vi "SaveDeviceHeader.vi"(0 "File Refnum in":refnum<file>, 1 "no. of arrays":i32, 3 "Array Lengths":i32, 5 "Filename":string, 7 "Run Number":i32, 9 "Array Titles":string, 11 "error in (no error)":errorcluster, 12 "Temperature":dbl, 13 "Humidity":dbl, 14 "Strip Segment":string) -> (4 "File Refnum out":refnum<file>, 6 "Header string":string, 10 "error out":errorcluster)   [LabVIEW 2018]
uses:
  globals/QC_RunInformation.vi
  InstrControl/InstrumentSetup.vi
  globals/QC_MeasurementSetup.vi
  InstrControl/LCRControl/LCRControl.lvclass
  <vilib>/regexp/Match Regular Expression.xnode
  InstrControl/InstrControl.lvclass
panel:
  out "File header":string
  out "File name":string
  out "Instr. conf.":string
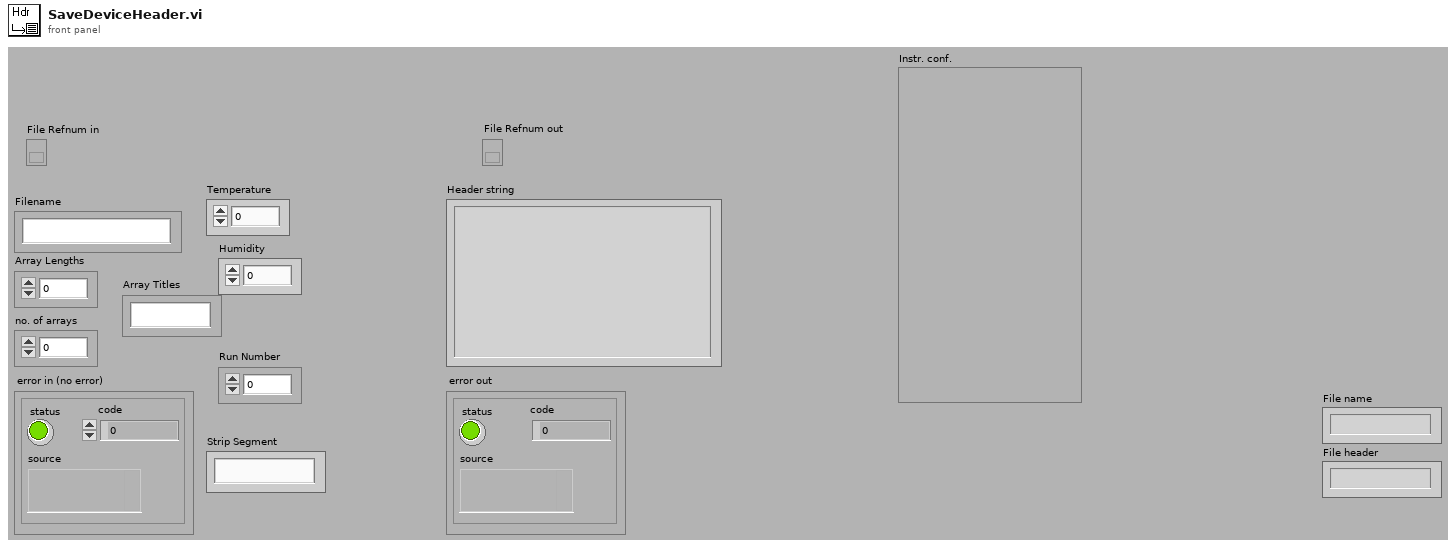
[diagram p1: front panel]
types:
  T1 = cluster{"Sensor Serial No.:":string, "Wafer:":string, "Batch:":string, "Manufacturer:":string, "Device Category:":string, "Database Serial No.:":string, "Date Initiated:":string, "Time Initiated:":string, "Test":string, "Probeplan used:":string, "End of Run Status":dbl, "End of Run comment:":string, "User:":string, "Vbias SMU":string, "LCR":string, "Test SMU":string, "Test DMM":string, "Comments":string, "Measurement results":cluster{"IV":string, "CV":string, "Cis":string, "Ris":string, "Stability":string, "PTP":string, "Striptest":string}}
  T2 = cluster{"Institute":string, "Manufacturers":string[], "Devices":string[], "Serialnumbers Lookup DB":string, "Data directory":string, "Backup & screenshot directory":string, "List of known users":string[], "Measurement switch not used":bool, "Measurement Switch":string, "DUT Switch":string, "Rseries IV [MOhm]":string, "Rshunt IV [MOhm]":string, "Rseries CV [MOhm]":string, "DC blocking Cap [µF]":string, "Rseries LCR [MOhm]":string, "Rseries stability [MOhm]":string, "Rshunt stability [MOhm]":string, "Rseries striptest bias [MOhm]":string, "Rseries strip pinhole [MOhm]":string}
  T3 = cluster{"Supply":refnum<class "SupplyControl.lvclass">, "LCR":refnum<class "LCRControl.lvclass">, "Arduino":refnum<class "ArduinoControl.lvclass">, "Measurement switch":refnum<class "Switching.lvclass">, "Initial Voltage [V]":dbl, "Final Voltage [V]":dbl, "Step Size [V]":dbl, "Step Interval [s]":i32, "Number Of Steps":u32, "Ramp down steps [V]":dbl, "Ramp down Interval [s]":i32, "Set Current Limit?":bool, "Current Limit [µA]":dbl, "Temperature Readout":enum16{"Read Arduino", "Enter manually"}, "Supply Name":string, "LCR Name":string, "V_depletion Limit [V]":dbl, "Measurement switch used?":bool}
  T4 = cluster{"RC Configuration":u16, "AC amplitude [V]":dbl, "AC frequency [Hz]":i32, "HP 4284A Configurations":cluster{"Consider OC":bool, "Consider SC":bool}}
  T5 = cluster{"Bias Supply":refnum<class "SupplyControl.lvclass">, "SMU":refnum<class "SupplyControl.lvclass">, "LCR":refnum<class "LCRControl.lvclass">, "ProbeStation":refnum<class "ProbeStationControl.lvclass">, "Arduino":refnum<class "ArduinoControl.lvclass">, "Measurement switch":refnum<class "Switching.lvclass">, "Probe Card Channels":i32, "Bias Voltage [V]":dbl, "First strip":i32, "Last strip":i32, "Base Voltage [V]":dbl, "Base Ramp Step [V]":dbl, "Base Ramp Interval [ms]":u32, "High Voltage [V]":dbl, "High Ramp Step [V]":dbl, "High Ramp Interval [ms]":u32, "AC frequency [Hz]":i32, "AC amplitude [V]":dbl, "RC Configuration":u16, "Single Needle":bool, "Temperature Readout":enum16{"Read Arduino", "Enter manually"}, "Fraction of good strips [%]":dbl, "Measurement switch used?":bool, "Matrix X Channels":cluster{"Mux1 C1":i32, "Mux1 C2":i32, "Mux2 C1":i32, "Mux2 C2":i32}, "Pinholes Y/N":bool, "Capacitance Y/N":bool, "Resistance Y/N":bool, "Bias Supply Name":string, "SMU Name":string, "LCR Name":string}
  T6 = cluster{"Supply":refnum<class "SupplyControl.lvclass">, "LCR":refnum<class "LCRControl.lvclass">, "Arduino":refnum<class "ArduinoControl.lvclass">, "Measurement switch":refnum<class "Switching.lvclass">, "Initial Voltage [V]":dbl, "Final Voltage [V]":dbl, "Step Size [V]":dbl, "Step Interval [s]":i32, "Number Of Steps":u32, "AC frequency [Hz]":i32, "RC Configuration":u16, "AC amplitude [V]":dbl, "Ramp down steps [V]":dbl, "Ramp down Interval [s]":i32, "Set Current Limit?":bool, "Current Limit [µA]":dbl, "Temperature Readout":enum16{"Read Arduino", "Enter manually"}, "Supply Name":string, "LCR Name":string, "C_is Limit [pF/cm]":dbl, "Measurement switch used?":bool}
  T7 = cluster{"Bias Supply":refnum<class "SupplyControl.lvclass">, "SMU":refnum<class "SupplyControl.lvclass">, "Arduino":refnum<class "ArduinoControl.lvclass">, "Initial Voltage [V]":dbl, "Final Voltage [V]":dbl, "Step Size [V]":dbl, "Step Interval [s]":i32, "Number Of Steps":u32, "Ramp down steps [V]":dbl, "Ramp down Interval [s]":i32, "Bias Voltage [V]":dbl, "Set Current Limit?":bool, "Current Limit [µA]":dbl, "Temperature Readout":enum16{"Read Arduino", "Enter manually"}, "Bias Supply Name":string, "SMU Name":string}
  T8 = cluster{"Supply":refnum<class "SupplyControl.lvclass">, "DMM":refnum<class "MultimeterControl.lvclass">, "DUT switch":refnum<class "Switching.lvclass">, "Arduino":refnum<class "ArduinoControl.lvclass">, "Measurement switch":refnum<class "Switching.lvclass">, "Voltage [V]":dbl, "Measurement Interval [s]":i32, "Test Duration":u32, "Ramp up steps [V]":dbl, "Ramp up Interval [s]":u32, "Ramp down steps [V]":dbl, "Ramp down Interval [s]":i32, "Set Current Limit?":bool, "Current Limit [µA]":dbl, "Temperature Readout":enum16{"Read Arduino", "Enter manually"}, "Supply Name":string, "DMM Name":string, "Maximum current fluctuation [%]":dbl, "Measurement switch used?":bool, "DUT switch used?":bool}
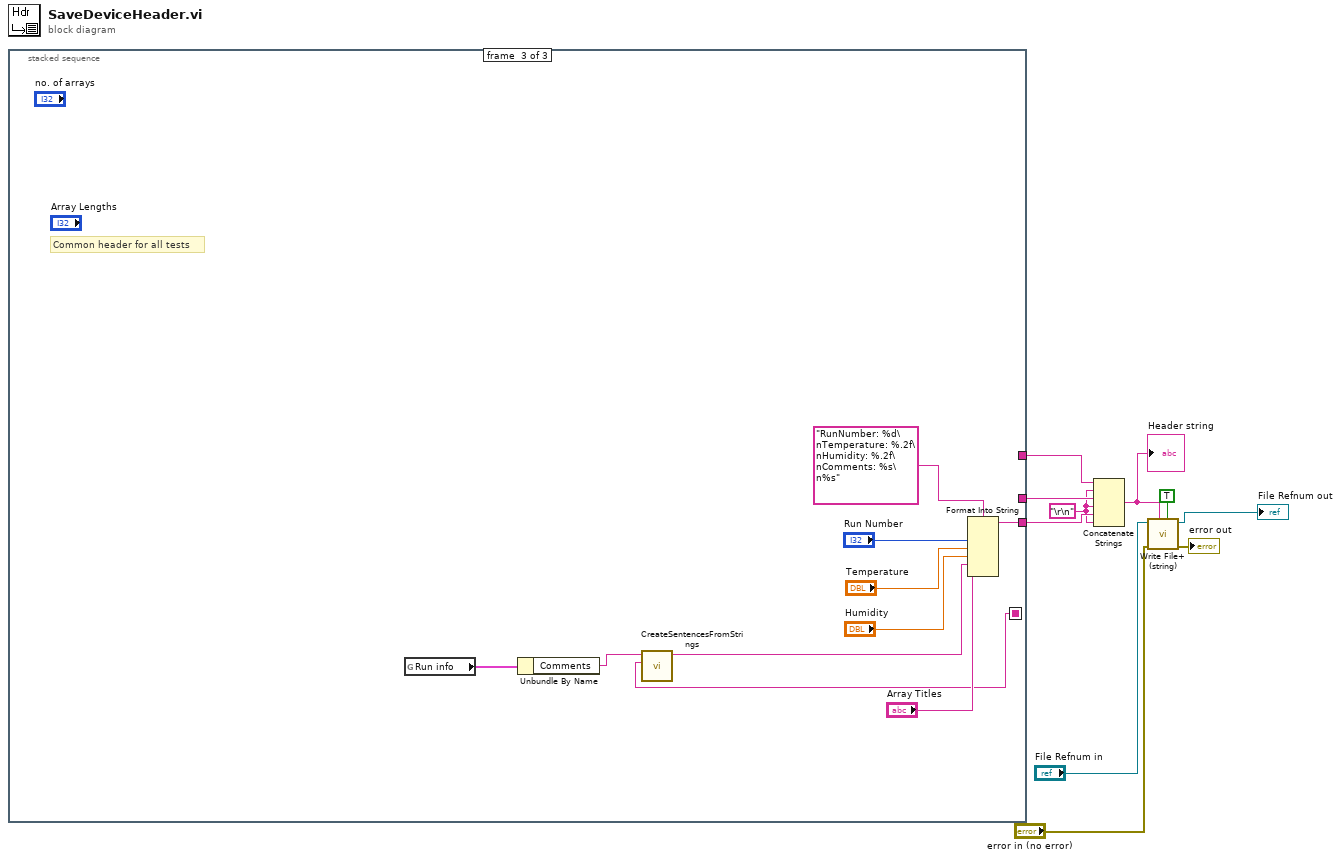
[diagram p0: block diagram]
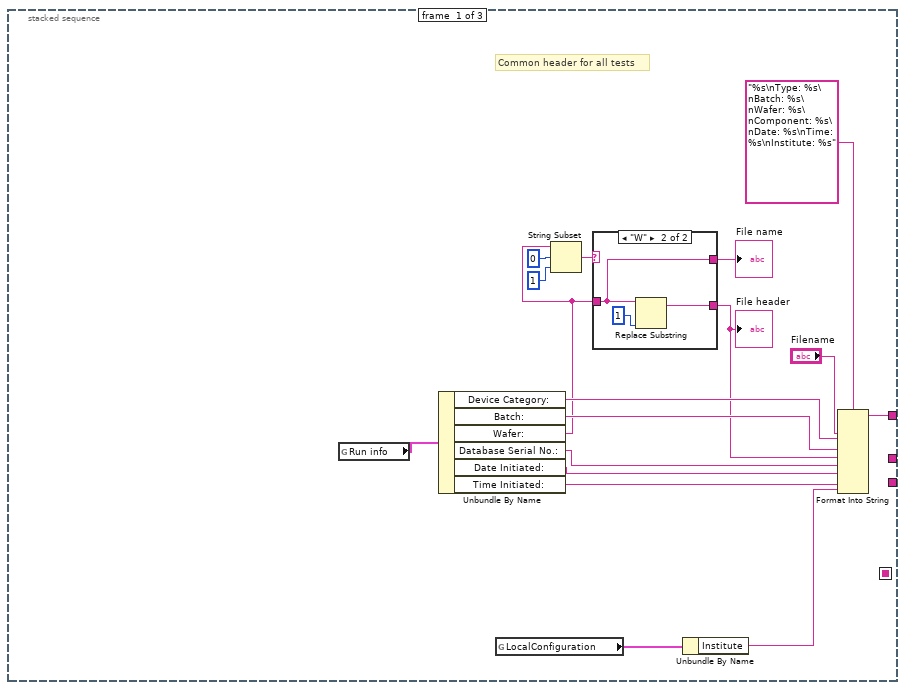
[diagram p2: hidden frame]
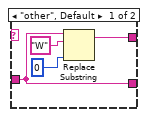
[diagram p3: hidden frame]
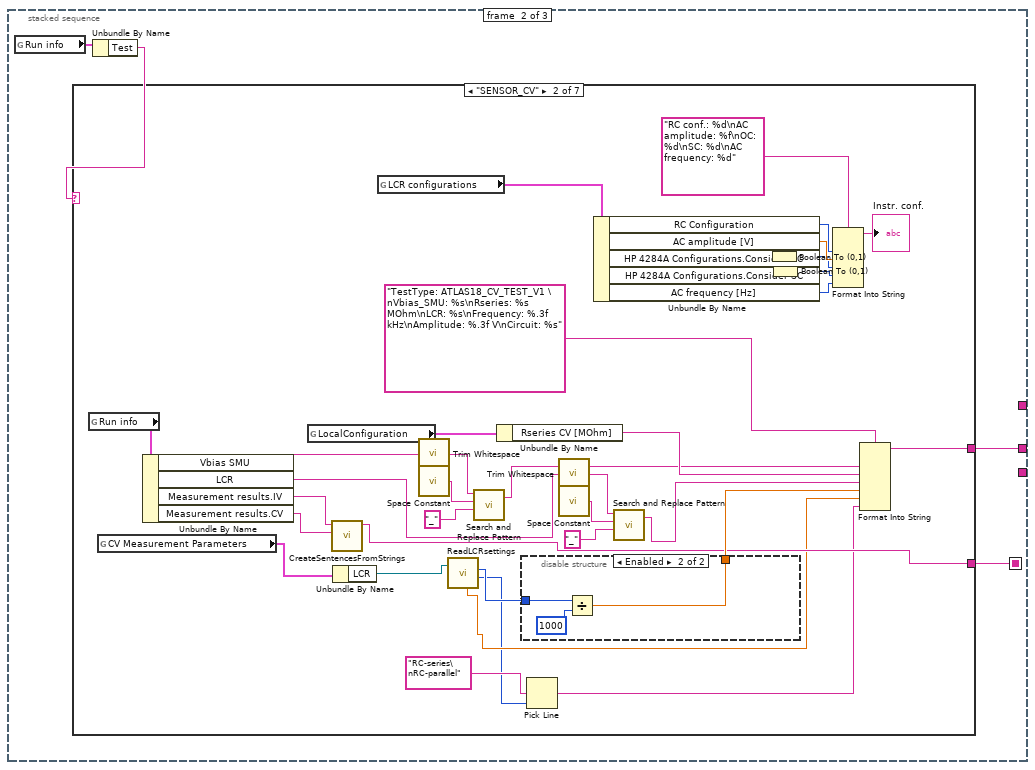
[diagram p4: hidden frame]
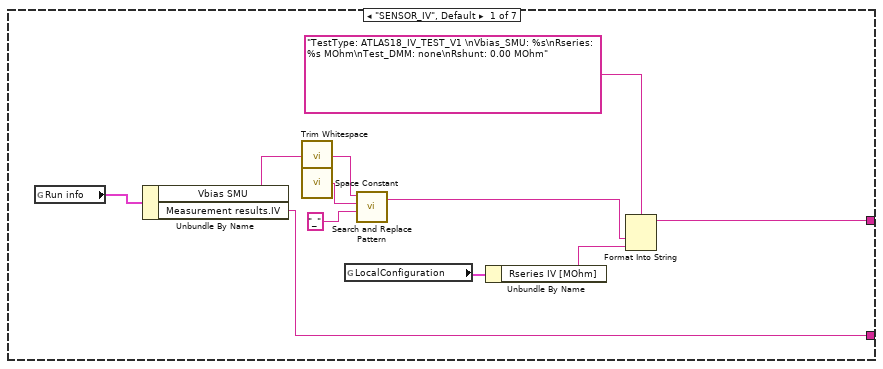
[diagram p5: hidden frame]
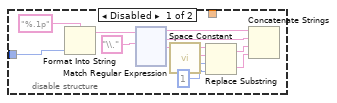
[diagram p6: hidden frame]
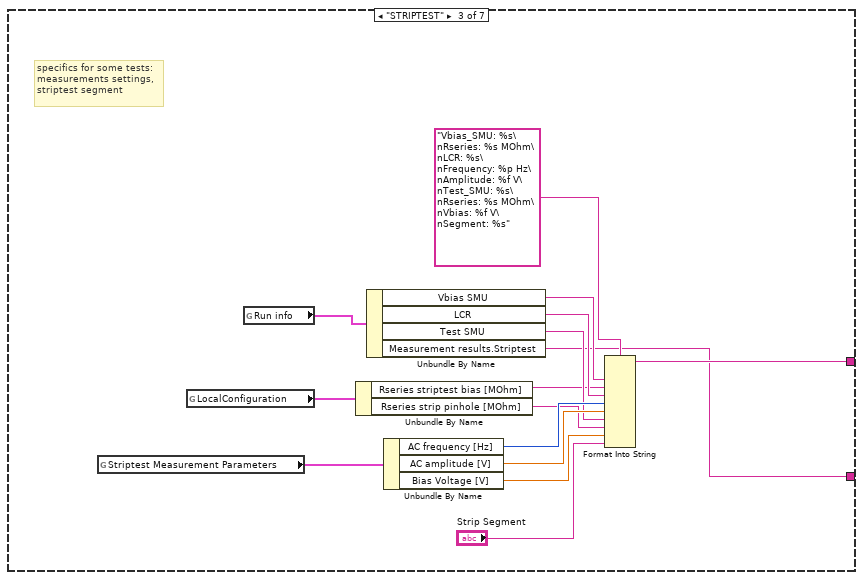
[diagram p7: hidden frame]
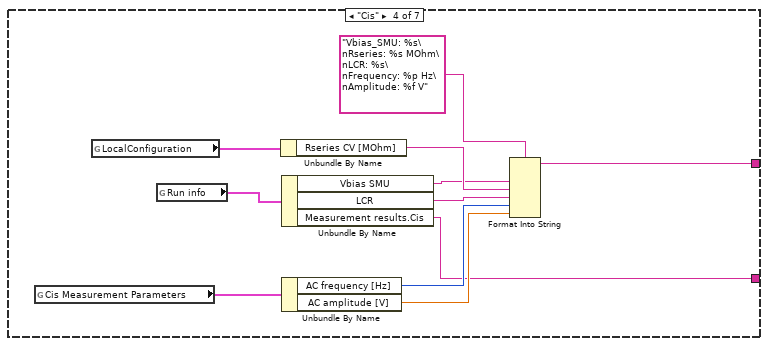
[diagram p8: hidden frame]
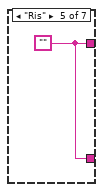
[diagram p9: hidden frame]
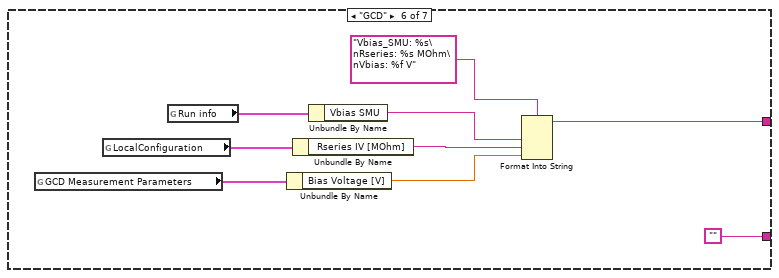
[diagram p10: hidden frame]
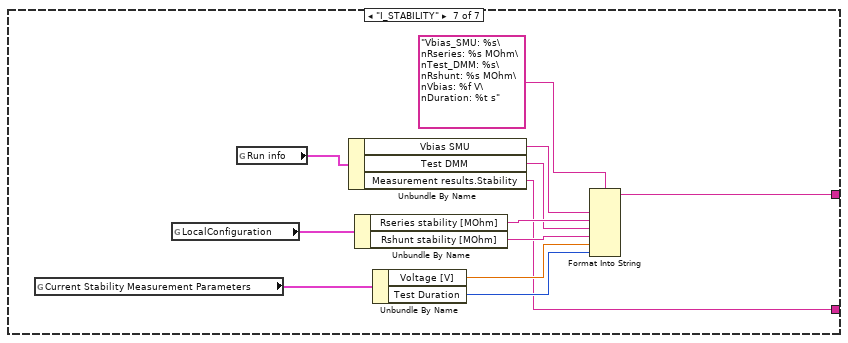
[diagram p11: hidden frame]
diagram:
  w2 = "\r\n"
  n1 = stacked-sequence {
    seq-local: [_ w35 _] -> [_ _ w263]
    tunnel: [_ w38 _] -> w6
    tunnel: [_ _ w267] -> w5
    tunnel: [w17 _ _] -> w4
    frame #0 {
      # "Common header for all tests"
      n2 = global read "QC_RunInformation.vi" "Run info"() -> (w19:T1)
      n3 = Unbundle By Name(w19) -> ("Device Category:"=w22:string, "Batch:"=w23:string, "Wafer:"=w12:string, "Database Serial No.:"=w24:string, "Date Initiated:"=w25:string, "Time Initiated:"=w26:string)
      n4 = global read "QC_RunInformation.vi" "LocalConfiguration"() -> (w18:T2)
      n5 = String Subset(string=w12, offset (0)=0, length (rest)=1 ("length (rest)")) -> (substring=w14:string)
      n6 = case shown="\"W\"" w14 {
        tunnel: [w29 w33] -> w13
        tunnel: w12 -> [w28 w33]
        tunnel: [w28 w34] -> w11
        frame "other", Default {
          n7 = Replace Substring(2:0 ("length (len. of substring)"), 4:"W" ("substring (\"\")"), 5:w28) -> (1:w29:string)  [unwired: 1 in, 1 out]
        }
        frame "W" {
          n8 = Replace Substring(2:1 ("length (len. of substring)"), 5:w33) -> (1:w34:string)  [unwired: 2 in, 1 out]
        }
      }
      "File name" <- w13
      "File header" <- w11
      n9 = Unbundle By Name(w18) -> ("Institute"=w27:string)
      n10 = Format Into String(format string="%s\nType: %s\nBatch: %s\nWafer: %s\nComponent: %s\nDate: %s\nTime: %s\nInstitute: %s", "Filename", w22, w23, w11, w24, w25, w26, w27) -> (resulting string=w17:string)  [unwired: 2 in, 1 out]
    }
    frame #1 {
      n11 = global read "QC_RunInformation.vi" "Run info"() -> (w37:T1)
      n12 = Unbundle By Name(w37) -> ("Test"=w36:string)
      n13 = case shown="\"SENSOR_CV\"" w36 {
        tunnel: [w45 w81 w225 w230 w240 w242 w257] -> w38
        tunnel: [w39 w58 w214 w229 w240 "" w250] -> w35
        frame "SENSOR_IV", Default {
          n14 = global read "QC_RunInformation.vi" "Run info"() -> (w48:T1)
          n15 = Unbundle By Name(w48) -> ("Vbias SMU"=w42:string, "Measurement results.IV"=w39:string)
          n16 = call <vilib>:"Trim Whitespace.vi"("string"=w42) -> ("trimmed string"=w41:string)  [unwired: 1 in]
          n17 = call <vilib>:"Space Constant.vi"() -> ("String"=w44:string)
          n18 = global read "QC_RunInformation.vi" "LocalConfiguration"() -> (w49:T2)
          n19 = call <vilib>:"Search and Replace Pattern.vi"("string"=w41, "regular expression (\"\")"=w44, "replace string (\"\")"="_" ("replace string (\"\")")) -> ("result string"=w40:string)  [unwired: 2 in, 1 out]
          n20 = Unbundle By Name(w49) -> ("Rseries IV [MOhm]"=w46:string)
          n21 = Format Into String(format string="TestType: ATLAS18_IV_TEST_V1 \nVbias_SMU: %s\nRseries: %s MOhm\nTest_DMM: none\nRshunt: 0.00 MOhm", w40, w46) -> (resulting string=w45:string)  [unwired: 2 in, 1 out]
        }
        frame "SENSOR_CV" {
          n22 = global read "QC_RunInformation.vi" "Run info"() -> (w84:T1)
          n23 = global read "QC_MeasurementSetup.vi" "CV Measurement Parameters"() -> (w53:T3)
          n24 = Unbundle By Name(w84) -> ("Vbias SMU"=w77:string, "LCR"=w72:string, "Measurement results.IV"=w60:string, "Measurement results.CV"=w59:string)
          n25 = global read "QC_RunInformation.vi" "LocalConfiguration"() -> (w85:T2)
          n26 = call "CreateSentencesFromStrings.vi"("String 2"=w59, "String 1"=w60) -> ("String 1. String 2"=w58:string)  [unwired: 8 in, 1 out]
          n27 = Unbundle By Name(w53) -> ("LCR"=w56:refnum<class "LCRControl.lvclass">)
          n28 = global read "InstrumentSetup.vi" "LCR configurations"() -> (w69:T4)
          n29 = call <vilib>:"Trim Whitespace.vi"("string"=w77) -> ("trimmed string"=w78:string)  [unwired: 1 in]
          n30 = call <vilib>:"Space Constant.vi"() -> ("String"=w80:string)
          n31 = call-dynamic "ReadLCRsettings.vi"("LCRControl in"=w56) -> ("RC Configuration"=w51:u16, "AC frequency [Hz]"=w55:i32, "AC amplitude [V]"=w54:sgl)  [unwired: 1 in, 2 out]
          n32 = call <vilib>:"Search and Replace Pattern.vi"("string"=w78, "regular expression (\"\")"=w80, "replace string (\"\")"="_" ("replace string (\"\")")) -> ("result string"=w76:string)  [unwired: 2 in, 1 out]
          n33 = Unbundle By Name(w85) -> ("Rseries CV [MOhm]"=w82:string)
          n34 = disable-structure shown="Enabled" {
            disable-tunnel: w55 -> [w86 w213]
            disable-tunnel: [_ w211] -> w70
            frame Disabled {
              w91 = 1 ("offset (0)")
              n35 = Format Into String(format string="%.1p", w86) -> (resulting string=w94:string)  [unwired: 2 in, 1 out]
              n36 = xnode "Match Regular Expression"("input string"=w94, "regular expression"="\\.") -> ("before match"=w90:string, "whole match"=w89:string, "after match"=w93:string)  [unwired: 4 in, 2 out]
              n37 = call <vilib>:"Space Constant.vi"() -> ("String"=w92:string)
              n38 = Replace Substring(2:w91, 3:w91, 4:w92, 5:w93) -> (0:w87:string, 1:w88:string)
              n39 = Concatenate Strings(w90, w89, w88, w87) -> ()  [unwired: 1 out]
            }
            frame Enabled {
              n40 = Divide(x=w213, y=1000) -> (x/y=w211:dbl)
            }
          }
          n41 = Pick Line(multi-line string="RC-series\nRC-parallel" ("string (\"\")"), line index=w51) -> (output string=w50:string)  [unwired: 1 in]
          n42 = call <vilib>:"Trim Whitespace.vi"("string"=w72) -> ("trimmed string"=w73:string)  [unwired: 1 in]
          n43 = call <vilib>:"Space Constant.vi"() -> ("String"=w75:string)
          n44 = Unbundle By Name(w69) -> ("RC Configuration"=w66:u16, "AC amplitude [V]"=w65:dbl, "HP 4284A Configurations.Consider OC"=w68:bool, "HP 4284A Configurations.Consider SC"=w67:bool, "AC frequency [Hz]"=w62:i32)
          n45 = call <vilib>:"Search and Replace Pattern.vi"("string"=w73, "regular expression (\"\")"=w75, "replace string (\"\")"="_" ("replace string (\"\")")) -> ("result string"=w71:string)  [unwired: 2 in, 1 out]
          n46 = Boolean To (0,1)(Boolean=w68) -> (0, 1=w64:i16)
          n47 = Boolean To (0,1)(Boolean=w67) -> (0, 1=w63:i16)
          n48 = Format Into String(format string="RC conf.: %d\nAC amplitude: %f\nOC: %d\nSC: %d\nAC frequency: %d", w66, w65, w64, w63, w62) -> (resulting string=→"Instr. conf.":string)  [unwired: 2 in, 1 out]
          n49 = Format Into String(format string="TestType: ATLAS18_CV_TEST_V1 \nVbias_SMU: %s\nRseries: %s MOhm\nLCR: %s\nFrequency: %.3f kHz\nAmplitude: %.3f V\nCircuit: %s", w76, w82, w71, w70, w54, w50) -> (resulting string=w81:string)  [unwired: 2 in, 1 out]
        }
        frame "STRIPTEST" {
          # "specifics for some tests:\nmeasurements settings,\nstriptest segment"
          n50 = global read "QC_MeasurementSetup.vi" "Striptest Measurement Parameters"() -> (w227:T5)
          n51 = global read "QC_RunInformation.vi" "LocalConfiguration"() -> (w218:T2)
          n52 = global read "QC_RunInformation.vi" "Run info"() -> (w228:T1)
          n53 = Unbundle By Name(w218) -> ("Rseries striptest bias [MOhm]"=w217:string, "Rseries strip pinhole [MOhm]"=w215:string)
          n54 = Unbundle By Name(w228) -> ("Vbias SMU"=w221:string, "LCR"=w220:string, "Test SMU"=w219:string, "Measurement results.Striptest"=w214:string)
          n55 = Unbundle By Name(w227) -> ("AC frequency [Hz]"=w224:i32, "AC amplitude [V]"=w223:dbl, "Bias Voltage [V]"=w216:dbl)
          n56 = Format Into String(format string="Vbias_SMU: %s\nRseries: %s MOhm\nLCR: %s\nFrequency: %p Hz\nAmplitude: %f V\nTest_SMU: %s\nRseries: %s MOhm\nVbias: %f V\nSegment: %s", w221, w217, w220, w224, w223, w219, w215, w216, "Strip Segment") -> (resulting string=w225:string)  [unwired: 2 in, 1 out]
        }
        frame "Cis" {
          n57 = global read "QC_MeasurementSetup.vi" "Cis Measurement Parameters"() -> (w239:T6)
          n58 = global read "QC_RunInformation.vi" "LocalConfiguration"() -> (w238:T2)
          n59 = global read "QC_RunInformation.vi" "Run info"() -> (w237:T1)
          n60 = Unbundle By Name(w238) -> ("Rseries CV [MOhm]"=w235:string)
          n61 = Unbundle By Name(w237) -> ("Vbias SMU"=w234:string, "LCR"=w233:string, "Measurement results.Cis"=w229:string)
          n62 = Unbundle By Name(w239) -> ("AC frequency [Hz]"=w232:i32, "AC amplitude [V]"=w231:dbl)
          n63 = Format Into String(format string="Vbias_SMU: %s\nRseries: %s MOhm\nLCR: %s\nFrequency: %p Hz\nAmplitude: %f V", w234, w235, w233, w232, w231) -> (resulting string=w230:string)  [unwired: 2 in, 1 out]
        }
        frame "Ris" {
          w240 = ""
        }
        frame "GCD" {
          n64 = global read "QC_MeasurementSetup.vi" "GCD Measurement Parameters"() -> (w244:T7)
          n65 = global read "QC_RunInformation.vi" "LocalConfiguration"() -> (w249:T2)
          n66 = global read "QC_RunInformation.vi" "Run info"() -> (w248:T1)
          n67 = Unbundle By Name(w244) -> ("Bias Voltage [V]"=w243:dbl)
          n68 = Unbundle By Name(w249) -> ("Rseries IV [MOhm]"=w246:string)
          n69 = Unbundle By Name(w248) -> ("Vbias SMU"=w245:string)
          n70 = Format Into String(format string="Vbias_SMU: %s\nRseries: %s MOhm\nVbias: %f V", w245, w246, w243) -> (resulting string=w242:string)  [unwired: 2 in, 1 out]
        }
        frame "I_STABILITY" {
          n71 = global read "QC_MeasurementSetup.vi" "Current Stability Measurement Parameters"() -> (w261:T8)
          n72 = global read "QC_RunInformation.vi" "LocalConfiguration"() -> (w260:T2)
          n73 = global read "QC_RunInformation.vi" "Run info"() -> (w259:T1)
          n74 = Unbundle By Name(w259) -> ("Vbias SMU"=w256:string, "Test DMM"=w254:string, "Measurement results.Stability"=w250:string)
          n75 = Unbundle By Name(w260) -> ("Rseries stability [MOhm]"=w255:string, "Rshunt stability [MOhm]"=w253:string)
          n76 = Unbundle By Name(w261) -> ("Voltage [V]"=w252:dbl, "Test Duration"=w251:u32)
          n77 = Format Into String(format string="Vbias_SMU: %s\nRseries: %s MOhm\nTest_DMM: %s\nRshunt: %s MOhm\nVbias: %f V\nDuration: %t s", w256, w255, w254, w253, w252, w251) -> (resulting string=w257:string)  [unwired: 2 in, 1 out]
        }
      }
    }
    frame #2 {
      # "Common header for all tests"
      n78 = global read "QC_RunInformation.vi" "Run info"() -> (w265:T1)
      n79 = Unbundle By Name(w265) -> ("Comments"=w264:string)
      n80 = call "CreateSentencesFromStrings.vi"("String 2"=w263, "String 1"=w264) -> ("String 1. String 2"=w262:string)  [unwired: 8 in, 1 out]
      n81 = Format Into String(format string="RunNumber: %d\nTemperature: %.2f\nHumidity: %.2f\nComments: %s\n%s", "Run Number", "Temperature", "Humidity", w262, "Array Titles") -> (resulting string=w267:string)  [unwired: 2 in, 1 out]
    }
  }
  n82 = Concatenate Strings(w4, w2, w6, w2, w5, w2) -> (w3:string)
  "Header string" <- w3
  n83 = call <vilib>:"Write File+ (string).vi"("convert eol? (no:F)"=TRUE, "string"=w3, "error in (no error)"="error in (no error)", "refnum"="File Refnum in") -> ("error out"=→"error out":errorcluster, "dup refnum"=→"File Refnum out":refnum<file>)  [unwired: 3 in, 1 out]
